vi "NormalizeAngle.vi"(1 "Angle":dbl) -> (0 "AngleFrom(0-360)":dbl)   [LabVIEW 2011]
panel:
  # "Reduces angle to between 0-360"
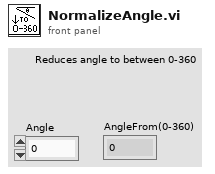
[diagram p1: front panel]
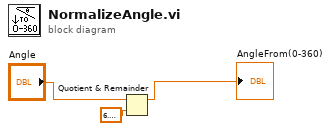
[diagram p0: block diagram]
diagram:
  n1 = Quotient & Remainder(x="Angle", y=6.283185307179586) -> (x-y*floor(x/y)=→"AngleFrom(0-360)":dbl)  [unwired: 1 out]
